vi "Stanford Research SR865 Data Capture.vi"() -> ()   [LabVIEW 2020]
doc: "Configures the data capture and then acquire all or parts of data capture buffer."
uses:
  Stanford Research SR865.lvlib
panel:
  out "Capture Buffer Contents":sgl[](array[numeric])
  in  "Data Length (0 kbytes)":i32
  in  "Data Offset (0 kbytes)":i32
  out "Data from Position":string
  out "Data Capture Amount(kilobytes)":dbl
  in  "Position (0: Oldest data from buffer)":i32
  in  "Stop Capture":bool
  out "Capture State Cluster":T1
  in  "Hardware Trigger State (0: OFF (immediately))":bool
  in  "Type (0: OneShot)":i32(ring) items=["OneShot", "Continuous"]
  in  "Capture Rate (0)":dbl
  in  "Capture Configuration (0: X)":i32(ring) items=["X", "X andY", "R and Theta", "X, Y, R and Theta"]
  in  "Capture Buffer Length (4 kbytes)":dbl=4.0
  in  "VISA resource name":refnum<visa-resource-name>
  # "(c) 2015 National Instruments.  ALL RIGHTS RESERVED."
  # "Capture Configuration"
  # "Data Position Configuration"
  # "Start Capture"
  # "Data Position Configuration"
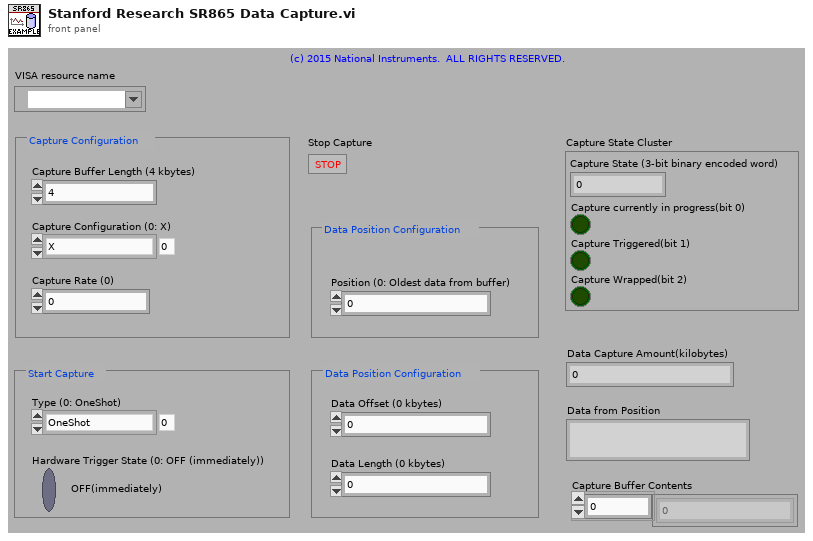
[diagram p1: front panel]
types:
  T1 = cluster{"Capture State (3-bit binary encoded word)":i32, "Capture currently in progress(bit 0)":bool, "Capture Triggered(bit 1)":bool, "Capture Wrapped(bit 2)":bool}
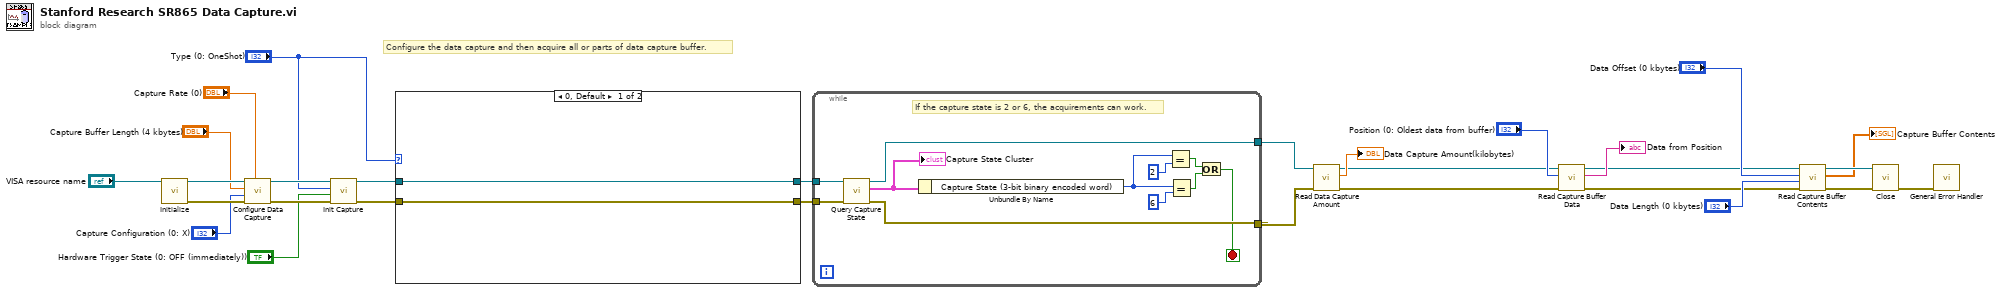
[diagram p0: block diagram]
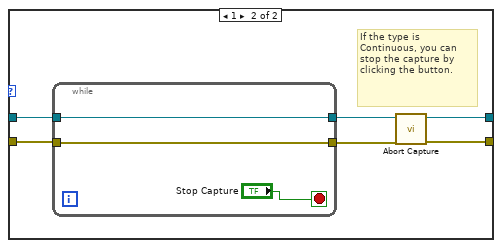
[diagram p2: hidden frame]
diagram:
  # "Configure the data capture and then acquire all or parts of data capture buffer."
  n1 = call "Initialize.vi"("VISA resource name"="VISA resource name") -> ("error out"=w27:errorcluster, "VISA resource name out"=w28:refnum<visa-resource-name>)  [unwired: 9 in]
  n2 = call "Configure Data Capture.vi"("Capture Rate (0)"="Capture Rate (0)", "error in (no error)"=w27, "Capture Configuration (0: X)"="Capture Configuration (0: X)", "Capture Buffer Length (4 kbytes)"="Capture Buffer Length (4 kbytes)", "VISA resource name"=w28) -> ("error out"=w22:errorcluster, "VISA resource name out"=w23:refnum<visa-resource-name>)  [unwired: 5 in]
  n3 = call "Init Capture.vi"("error in (no error)"=w22, "Hardware Trigger State (0: OFF (immediately))"="Hardware Trigger State (0: OFF (immediately))", "Type (0: OneShot)"="Type (0: OneShot)", "VISA resource name"=w23) -> ("error out"=w13:errorcluster, "VISA resource name out"=w14:refnum<visa-resource-name>)  [unwired: 6 in]
  n4 = case shown="0, Default" "Type (0: OneShot)" {
    tunnel: [w31 w34] -> w12
    tunnel: w14 -> [w31 w37]
    tunnel: [w30 w33] -> w11
    tunnel: w13 -> [w30 w35]
    frame 0, Default {
    }
    frame 1 {
      # "If the type is Continuous, you can stop the capture by clicking the button."
      n5 = while {
        tunnel: w37 -> [w40]
        tunnel: [w40] -> w36
        tunnel: w35 -> [w38]
        tunnel: [w38] -> w32
        stop <- "Stop Capture" stop-if-true
      }
      n6 = call "Abort Capture.vi"("error in (no error)"=w32, "VISA resource name"=w36) -> ("error out"=w33:errorcluster, "VISA resource name out"=w34:refnum<visa-resource-name>)  [unwired: 8 in]
    }
  }
  n7 = while {
    tunnel: w12 -> [w51]
    tunnel: w11 -> [w50]
    tunnel: [w47] -> w10
    tunnel: [w46] -> w9
    stop <- w41 stop-if-true
    # "If the capture state is 2 or 6, the acquirements can work."
    n8 = call "Query Capture State.vi"("error in (no error)"=w50, "VISA resource name"=w51) -> ("error out"=w46:errorcluster, "Capture State Cluster"=w49:T1, "VISA resource name out"=w47:refnum<visa-resource-name>)  [unwired: 7 in]
    "Capture State Cluster" <- w49
    n9 = Unbundle By Name(w49) -> ("Capture State (3-bit binary encoded word)"=w45:i32)
    n10 = Equal?(x=w45, y=2) -> (x = y?=w43:bool)
    n11 = Equal?(x=w45, y=6) -> (x = y?=w42:bool)
    n12 = Or(x=w43, y=w42) -> (x .or. y?=w41:bool)
  }
  n13 = call "Read Data Capture Amount.vi"("error in (no error)"=w9, "VISA resource name"=w10) -> ("error out"=w7:errorcluster, "Data Capture Amount(kilobytes)"=→"Data Capture Amount(kilobytes)":dbl, "VISA resource name out"=w8:refnum<visa-resource-name>)  [unwired: 7 in]
  n14 = call "Read Capture Buffer Data.vi"("error in (no error)"=w7, "Position (0: Oldest data from buffer)"="Position (0: Oldest data from buffer)", "VISA resource name"=w8) -> ("error out"=w5:errorcluster, "Data from Position"=→"Data from Position":string, "VISA resource name out"=w6:refnum<visa-resource-name>)  [unwired: 6 in]
  n15 = call "Read Capture Buffer Contents.vi"("error in (no error)"=w5, "Data Length (0 kbytes)"="Data Length (0 kbytes)", "Data Offset (0 kbytes)"="Data Offset (0 kbytes)", "VISA resource name"=w6) -> ("error out"=w3:errorcluster, "Capture Buffer Contents"=→"Capture Buffer Contents":sgl[], "VISA resource name out"=w4:refnum<visa-resource-name>)  [unwired: 5 in]
  n16 = call "Close.vi"("error in (no error)"=w3, "VISA resource name"=w4) -> ("error out"=w2:errorcluster)  [unwired: 9 in]
  n17 = call <vilib>:"General Error Handler.vi"("error in (no error)"=w2) -> ()  [unwired: 10 in, 5 out]
